vi "init_virtualSpectrometer.vi"(0 "idxSpectr":u16, 2 "model":T1, 5 "error in (no error)":errorcluster) -> (14 "idxSpectr copy":u16, 16 "OSA series":enum16{"OSA200", "OSA300", "UNKNOWN"}(ring), 19 "error out":errorcluster)   [LabVIEW 2010, in "OSA.lvclass"]
doc: "Lower level init routine, higher level routines will be sufficient in most cases."
uses:
  OSA.lvclass
  _misc/Thorlabs_FTS_misc.llb/OSA_virtualModel.ctl
  FTSLib.dll
  OSA20X_misc.lvlib
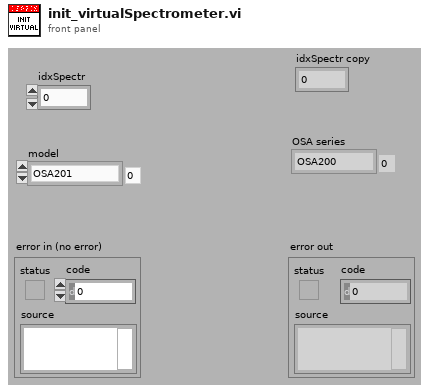
[diagram p1: front panel]
types:
  T1 = typedef "OSA20X_misc.lvlib/OSA_virtualModel.ctl" = enum16{"OSA201", "OSA201C", "OSA202", "OSA202C", "OSA203", "OSA203B", "OSA203C", "OSA205", "OSA205C", "REDSTONE301", "REDSTONE305"}
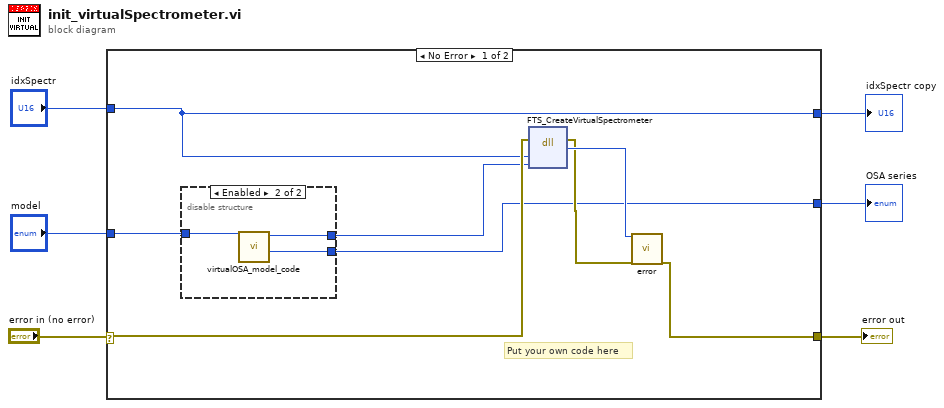
[diagram p0: block diagram]
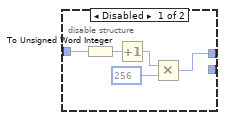
[diagram p2: hidden frame]
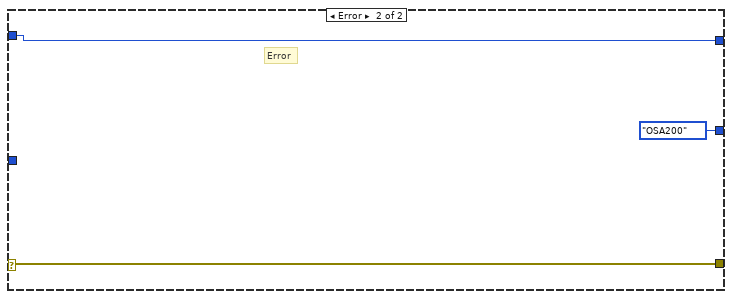
[diagram p3: hidden frame]
diagram:
  n1 = case shown="No Error" "error in (no error)" {
    selector: "error in (no error)" -> [w14 w25]
    tunnel: [w8 w25] -> w6
    tunnel: "idxSpectr" -> [w13 w24]
    tunnel: "model" -> [w12 _]
    tunnel: [w13 w24] -> w2
    tunnel: [w7 enum16{"OSA200", "OSA300", "UNKNOWN"}."OSA200" ("OSA series")] -> w1
    frame No Error {
      # "Put your own code here"
      n2 = disable-structure shown="Enabled" {
        disable-tunnel: w12 -> [w19 w22]
        disable-tunnel: [w16 w21] -> w11
        disable-tunnel: [_ w20] -> w7
        frame Disabled {
          n3 = To Unsigned Word Integer(number=w19) -> (unsigned 16bit integer=w17:u16)
          n4 = Increment(x=w17) -> (x+1=w15:u16)
          n5 = Multiply(x=w15, y=u16 256) -> (x*y=w16:u16)
        }
        frame Enabled {
          n6 = call "virtualOSA_model_code.vi"("virtual OSA model"=w22) -> ("OSA series"=w20:enum16{"OSA200", "OSA300", "UNKNOWN"}, "virtualOSA code"=w21:u16)  [unwired: 9 in]
        }
      }
      n7 = dll-call lib="FTSLib.dll" fn="FTS_CreateVirtualSpectrometer"(error in=w14, "idxSpectr"=w13, "model"=w11) -> (error out=w9:errorcluster, "return type"=w10:i32)  [unwired: 4 in, 1 out]
      n8 = call "error.vi"("result code"=w10, "error in (no error)"=w9) -> ("error out"=w8:errorcluster)  [unwired: 15 in, 2 out]
    }
    frame Error {
      # "Error"
    }
  }
  "error out" <- w6
  "idxSpectr copy" <- w2
  "OSA series" <- w1
